vi "FlattenSaveClassData.vi"(8 "error in":errorcluster, 10 "Class Data File Path":path, 11 "TestCase in":refnum<class "TestCase.lvclass">) -> (0 "error out":errorcluster, 3 "TestCase out":refnum<class "TestCase.lvclass">)   [LabVIEW 2027, in "VeriStandTestUtilities.lvlib"]
uses:
  VeriStandTestUtilities.lvlib
  <vilib>/addons/_JKI Toolkits/VI Tester/TestCase.llb/TestCase.lvclass
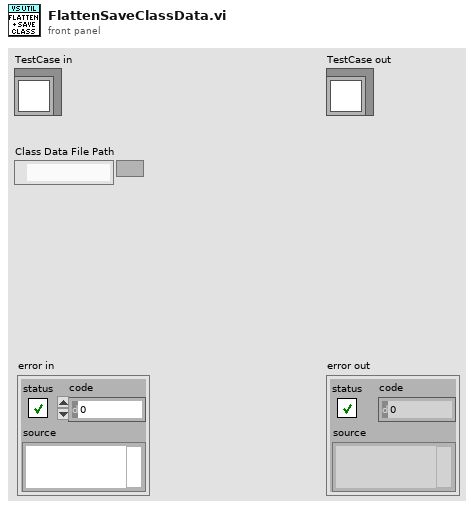
[diagram p1: front panel]
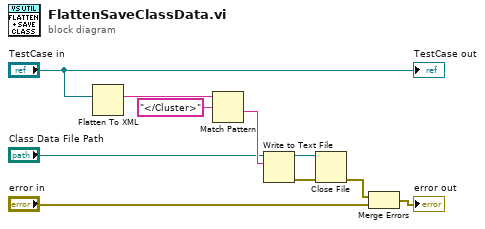
[diagram p0: block diagram]
diagram:
  n1 = Flatten To XML(6:"TestCase in") -> (2:w10:string)
  n2 = Match Pattern(string=w10, regular expression="</Cluster>") -> (after substring=w8:string)  [unwired: 1 in, 3 out]
  n3 = Write to Text File(file (use dialog)="Class Data File Path", text=w8) -> (refnum out=w3:refnum<file>, error out=w7:errorcluster)  [unwired: 2 in, 1 out]
  n4 = Close File(refnum=w3, error in=w7) -> (error out=w6:errorcluster)  [unwired: 1 out]
  n5 = Merge Errors(w6, "error in") -> (→"error out":errorcluster)
  "TestCase out" <- "TestCase in"
